vi "solar_misc LVClass List.vi"() -> (0 "All LVClasses in Memory":string[](array[string]))   [LabVIEW 2018]
doc: "This VI lists all LabVIEW Classes (*.lvclass) in memory.\n\nCreated By: Ryan Pacini\nDate: 5/28/2016"
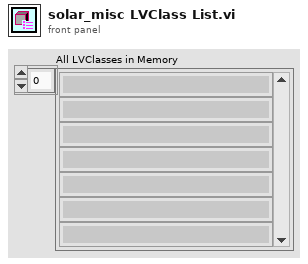
[diagram p1: front panel]
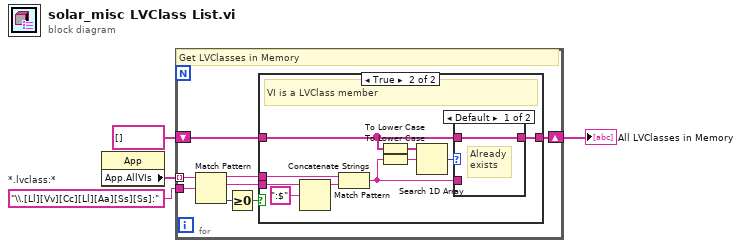
[diagram p0: block diagram]
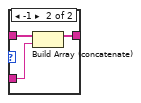
[diagram p3: hidden frame]
diagram:
  w2 = "\\.[Ll][Vv][Cc][Ll][Aa][Ss][Ss]:"  # *.lvclass:*
  n1 = property class="App"() -> ("App.AllVIs"=w4:string[])  [unwired: 2 in, 2 out]
  n2 = for {
    tunnel: w4 -> [w11] mode=indexing
    shift-right: [w8] -> w1
    shift-left: string[] [] -> [w7]
    tunnel: w2 -> [w10]
    # "Get LVClasses in Memory"
    n3 = Match Pattern(string=w11, regular expression=w10) -> (before substring=w6:string, match substring=w5:string, offset past match=w12:i32)  [unwired: 1 in, 1 out]
    n4 = Greater Or Equal To 0?(x=w12) -> (x >= 0?=w9:bool)
    n5 = case shown="True" w9 {
      tunnel: [w13 w22] -> w8
      tunnel: w7 -> [w13 w18]
      tunnel: w6 -> [_ w23]
      tunnel: w5 -> [_ w21]
      frame False {
        # "VI is not a LVClass member"
      }
      frame True {
        # "VI is a LVClass member"
        n6 = Match Pattern(string=w21, regular expression=":$") -> (before substring=w19:string)  [unwired: 1 in, 3 out]
        n7 = Concatenate Strings(w23, w19) -> (w15:string)
        n8 = To Lower Case(string=w18) -> (all lower case string=w17:string[])
        n9 = To Lower Case(string=w15) -> (all lower case string=w16:string)
        n10 = Search 1D Array(1D array=w17, element=w16) -> (index of element=w14:i32)  [unwired: 1 in]
        n11 = case shown="Default" w14 {
          tunnel: [w24 w27] -> w22
          tunnel: w18 -> [w24 w26]
          tunnel: w15 -> [_ w25]
          frame Default {
            # "Already\nexists"
          }
          frame -1 {
            n12 = Build Array (concatenate)(w26, w25) -> (w27:string[])
          }
        }
      }
    }
  }
  "All LVClasses in Memory" <- w1
